vi "encoder.vi"() -> ()   [LabVIEW 2019]
uses:
  <vilib>/Rock Robotics/SystemInterfaces/DIO/FPGA_DIOChannel.ctl
  <vilib>/Rock Robotics/WPI/Counter/WPI_CounterDigitalInputToDigitalSource.vi
  <vilib>/Rock Robotics/SystemInterfaces/AI/FPGA_AIChannel.ctl
panel:
  out "Normalized Value":dbl
  out "Switch":bool
  out "Stopped":bool
  out "Rate":dbl
  out "Direction":bool
  out "Distance":dbl
  in  "stop":bool
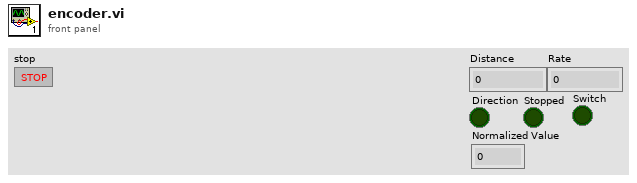
[diagram p1: front panel]
types:
  T1 = typedef "FPGA_AIChannel.ctl" = enum8{"AI 0", "AI 1", "AI 2", "AI 3", "AI MXP 0", "AI MXP 1", "AI MXP 2", "AI MXP 3", "Invalid"}
  T2 = typedef "FPGA_DIOChannel.ctl" = enum8{"DIO 0", "DIO 1", "DIO 2", "DIO 3", "DIO 4", "DIO 5", "DIO 6", "DIO 7", "DIO 8", "DIO 9", "DIO MXP 0", "DIO MXP 1", "DIO MXP 2", "DIO MXP 3", "DIO MXP 4", "DIO MXP 5", "DIO MXP 6", "DIO MXP 7", "DIO MXP 8", "DIO MXP 9", "DIO MXP 10", "DIO MXP 11", "DIO MXP 12", "DIO MXP 13", "DIO MXP 14", "DIO MXP 15", "SPI Port CS1", "SPI Port CS2", "SPI Port CS3", "SPI Port MISO", "SPI Port MOSI", "Invalid"}
  T3 = typedef "WPI_DigitalInputDevRef.ctl" = cluster{"DevStatus":errorcluster, "DIO Channel":T2}
  T4 = typedef "WPI_PotentiometerDevRef.ctl" = cluster{"DevStatus":errorcluster, "Analog Channel":T1, "Invert Output":bool}
  T5 = typedef "FPGA_CounterEncoderSourceConvertionLVSourceType.ctl" = cluster{"DevStatus":errorcluster, "AnalogTriggerMode?":bool, "DigitalMode":cluster{"DIO Channel":T6}, "AnalogTriggerMode":cluster{"AnalogTriggerIndex":T7, "OutputType":T8}}
  T6 = typedef "FPGA_DIODigitalSourceChannel.ctl" = enum8{"DIO 0", "DIO 1", "DIO 2", "DIO 3", "DIO 4", "DIO 5", "DIO 6", "DIO 7", "DIO 8", "DIO 9", "DIO MXP 0", "DIO MXP 1", "DIO MXP 2", "DIO MXP 3", "DIO MXP 4", "DIO MXP 5", "DIO MXP 6", "DIO MXP 7", "DIO MXP 8", "DIO MXP 9", "DIO MXP 10", "DIO MXP 11", "DIO MXP 12", "DIO MXP 13", "DIO MXP 14", "DIO MXP 15", "SPI Port CS1", "SPI Port CS2", "SPI Port CS3", "SPI Port MISO", "SPI Port MOSI", "Disabled"}
  T7 = typedef "FPGA_AnalogTriggerIndex.ctl" = enum8{"Trig 0", "Trig 1", "Trig 2", "Trig 3", "Trig 4", "Trig 5", "Trig 6", "Trig 7", "Invalid"}
  T8 = typedef "FPGA_AnalogTriggerOutType.ctl" = enum16{"InWindow", "TriggerState", "Rising", "Falling"}
  T9 = typedef "WPI_EncoderDevRef.ctl" = cluster{"DevStatus":errorcluster, "EncoderIndex":T10, "CounterIndex":T11, "DistancePerCount":dbl, "Decoding Type":T12}
  T10 = typedef "FPGA_EncoderIdx.ctl" = enum8{"Enc 0", "Enc 1", "Enc 2", "Enc 3", "Enc 4", "Enc 5", "Enc 6", "Enc 7", "Invalid"}
  T11 = typedef "FPGA_CounterCtrSystemIndex.ctl" = enum8{"Ctr 0", "Ctr 1", "Ctr 2", "Ctr 3", "Ctr 4", "Ctr 5", "Ctr 6", "Ctr 7", "Invalid"}
  T12 = typedef "WPI_EncoderType.ctl" = enum16{"1x", "2x", "4x"}
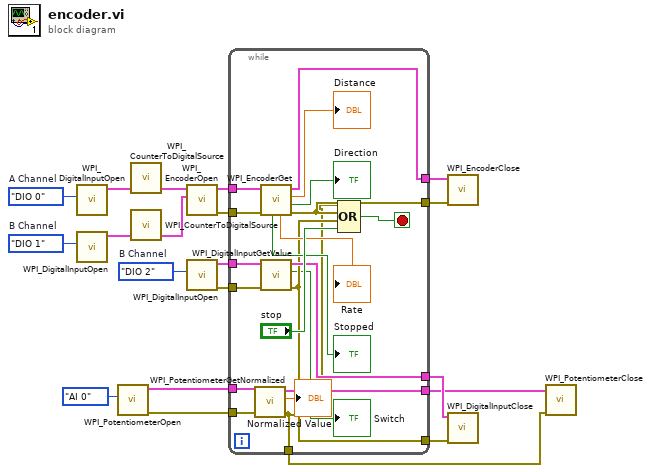
[diagram p0: block diagram]
diagram:
  w14 = FPGA_DIOChannel."DIO 2"  # B Channel
  w20 = FPGA_DIOChannel."DIO 1"  # B Channel
  w19 = FPGA_DIOChannel."DIO 0"  # A Channel
  n1 = call <vilib>:"WPI_DigitalInputOpen.vi"("DIO Channel"=w19) -> ("DigitalInputDevRef"=w16:T3)  [unwired: 1 in, 9 out]
  n2 = call <vilib>:"WPI_DigitalInputOpen.vi"("DIO Channel"=w20) -> ("DigitalInputDevRef"=w17:T3)  [unwired: 1 in, 9 out]
  n3 = call <vilib>:"WPI_PotentiometerOpen.vi"("Analog Channel"=FPGA_AIChannel."AI 0") -> ("error out"=w3:errorcluster, "PotDevRef"=w4:T4)  [unwired: 9 in]
  n4 = call-poly <vilib>:"WPI_CounterToDigitalSource.vi"("DigitalInputDevRef"=w16) -> ("Digital Source"=w15:T5)  [unwired: 6 out]
  n5 = call-poly <vilib>:"WPI_CounterToDigitalSource.vi"("DigitalInputDevRef"=w17) -> ("Digital Source"=w18:T5)  [unwired: 6 out]
  n6 = call <vilib>:"WPI_EncoderOpen.vi"("BSource"=w18, "ASource"=w15) -> ("error out"=w10:errorcluster, "EncoderDevRef"=w13:T9)  [unwired: 6 in, 2 out]
  n7 = call <vilib>:"WPI_DigitalInputOpen.vi"("DIO Channel"=w14) -> ("error out"=w11:errorcluster, "DigitalInputDevRef"=w12:T3)  [unwired: 1 in, 8 out]
  n8 = while {
    tunnel: w13 -> [w39]
    tunnel: w12 -> [w37]
    tunnel: w11 -> [w38]
    tunnel: w10 -> [w32]
    tunnel: [w30] -> w9
    tunnel: [w29] -> w8
    tunnel: [w28] -> w7
    tunnel: [w27] -> w6
    tunnel: w4 -> [w25]
    tunnel: w3 -> [w24]
    tunnel: [w23] -> w2
    tunnel: [w22] -> w1
    stop <- w31 stop-if-true
    n9 = call <vilib>:"WPI_PotentiometerGetNormalized.vi"("error in"=w24, "PotDevRef"=w25) -> ("error out"=w22:errorcluster, "Normalized Value"=→"Normalized Value":dbl, "PotDevRef"=w23:T4)  [unwired: 7 in]
    n10 = call <vilib>:"WPI_EncoderGet.vi"("error in (no error)"=w32, "EncoderDevRef"=w39) -> ("error out"=w29:errorcluster, "Direction"=→"Direction":bool, "Distance"=→"Distance":dbl, "EncoderDevRef"=w30:T9, "Rate"=→"Rate":dbl, "Stopped"=→"Stopped":bool)  [unwired: 4 in]
    n11 = call <vilib>:"WPI_DigitalInputGetValue.vi"("error in (no error)"=w38, "DigitalInputDevRef"=w37) -> ("error out"=w27:errorcluster, "Value"=→"Switch":bool, "DigitalInputDevRef"=w28:T3)  [unwired: 7 in]
    n12 = Compound Arithmetic op=OR(w22, w29, w27, "stop") -> (w31:bool)
  }
  n13 = call <vilib>:"WPI_EncoderClose.vi"("error in (no error)"=w8, "EncoderDevRef"=w9) -> ()  [unwired: 9 in, 1 out]
  n14 = call <vilib>:"WPI_DigitalInputClose.vi"("error in (no error)"=w6, "DigitalInputDevRef"=w7) -> ()  [unwired: 9 in, 1 out]
  n15 = call <vilib>:"WPI_PotentiometerClose.vi"("error in"=w1, "PotDevRef"=w2) -> ()  [unwired: 9 in, 1 out]
